vi "Pemutation_subvi.vi"() -> ()   [LabVIEW 2015]
panel:
  out "nCr":i32
  out "nPr":i32
  in  "R":i32
  in  "N":i32
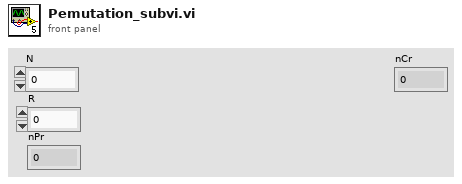
[diagram p1: front panel]
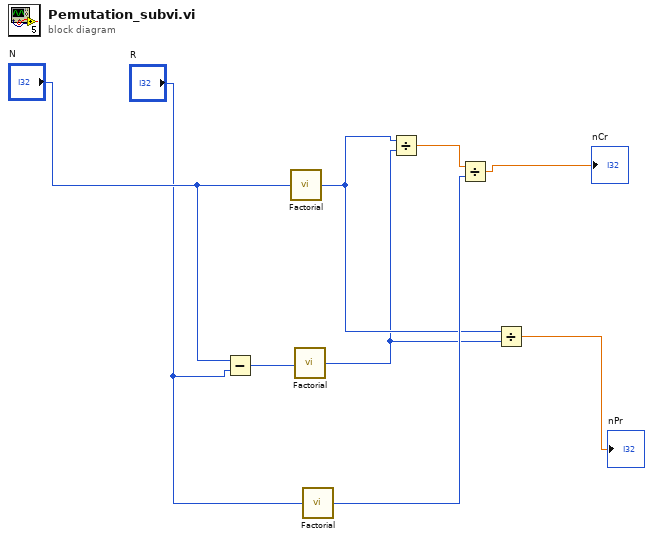
[diagram p0: block diagram]
diagram:
  n1 = Subtract(x="N", y="R") -> (x-y=w7:i32)
  n2 = call "Factorial.vi"("Input_num"="N") -> ("Numeric"=w3:i32)
  n3 = call "Factorial.vi"("Input_num"=w7) -> ("Numeric"=w2:i32)
  n4 = call "Factorial.vi"("Input_num"="R") -> ("Numeric"=w5:i32)
  n5 = Divide(x=w3, y=w2) -> (x/y=w6:dbl)
  n6 = Divide(x=w6, y=w5) -> (x/y=→"nCr":dbl)
  n7 = Divide(x=w3, y=w2) -> (x/y=→"nPr":dbl)
